vi "Version Compatibility Check.vi"(9 "Allow Equal?":bool, 10 "Old Version":string="1.0.0", 11 "New Version":string="1.0.0") -> (2 "Incompatible?":bool, 3 "Invalid Format?":bool)   [LabVIEW 2014]
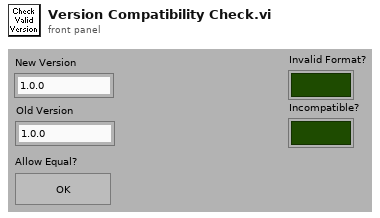
[diagram p1: front panel]
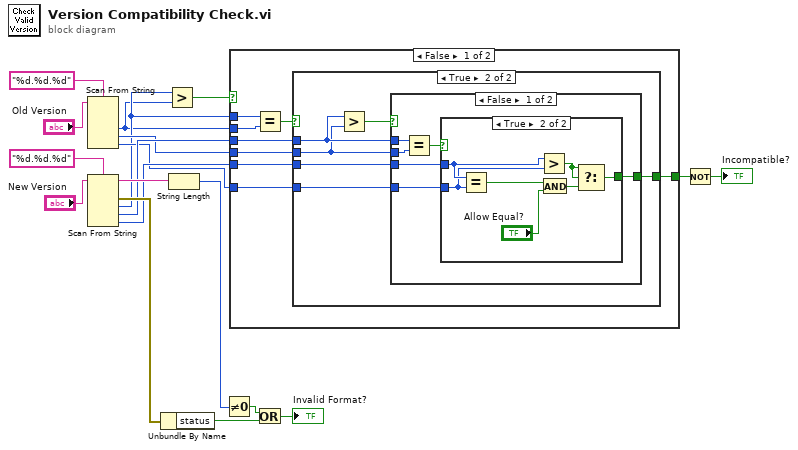
[diagram p0: block diagram]
diagram:
  n1 = Scan From String(format string="%d.%d.%d", input string="Old Version") -> (output 1=w3:i32, output 2=w8:i32, output 3=w6:i32)  [unwired: 5 in, 3 out]
  n2 = Scan From String(format string="%d.%d.%d", input string="New Version") -> (remaining string=w14:string, error out=w17:errorcluster, output 1=w4:i32, output 2=w9:i32, output 3=w7:i32)  [unwired: 5 in, 1 out]
  n3 = Unbundle By Name(w17) -> ("status"=w11:bool)
  n4 = Greater?(x=w4, y=w3) -> (0:w5:bool)
  n5 = String Length(string=w14) -> (length=w13:i32)
  n6 = Not Equal To 0?(x=w13) -> (x != 0?=w12:bool)
  n7 = case shown="False" w5 {
    selector: w5 -> [_ w50]
    tunnel: [w24 w50] -> w2
    tunnel: w4 -> [w27 _]
    tunnel: w3 -> [w26 _]
    tunnel: w9 -> [w23 _]
    tunnel: w7 -> [w21 _]
    tunnel: w8 -> [w22 _]
    tunnel: w6 -> [w20 _]
    frame False {
      n8 = Equal?(x=w27, y=w26) -> (x = y?=w25:bool)
      n9 = case shown="True" w25 {
        selector: w25 -> [w28 _]
        tunnel: [w28 w33] -> w24
        tunnel: w23 -> [_ w32]
        tunnel: w22 -> [_ w31]
        tunnel: w21 -> [_ w30]
        tunnel: w20 -> [_ w29]
        frame False {
        }
        frame True {
          n10 = Greater?(x=w32, y=w31) -> (0:w34:bool)
          n11 = case shown="False" w34 {
            selector: w34 -> [_ w49]
            tunnel: [w37 w49] -> w33
            tunnel: w32 -> [w40 _]
            tunnel: w31 -> [w39 _]
            tunnel: w30 -> [w36 _]
            tunnel: w29 -> [w35 _]
            frame False {
              n12 = Equal?(x=w40, y=w39) -> (x = y?=w38:bool)
              n13 = case shown="True" w38 {
                selector: w38 -> [w41 _]
                tunnel: [w41 w42] -> w37
                tunnel: w36 -> [_ w48]
                tunnel: w35 -> [_ w47]
                frame False {
                }
                frame True {
                  n14 = Equal?(x=w48, y=w47) -> (x = y?=w45:bool)
                  n15 = Greater?(x=w48, y=w47) -> (0:w46:bool)
                  n16 = And(x=w45, y="Allow Equal?") -> (x .and. y?=w43:bool)
                  n17 = Select(t=w46, s=w46, f=w43) -> (s? t:f=w42:bool)
                }
              }
            }
            frame True {
            }
          }
        }
      }
    }
    frame True {
    }
  }
  n18 = Or(x=w12, y=w11) -> (x .or. y?=→"Invalid Format?":bool)
  n19 = Not(x=w2) -> (.not. x?=→"Incompatible?":bool)
